vi "LinearSystemSim_setInput.vi"(9 "Battery_Volts":dbl=12.0, 10 "Input":T1, 11 "in LinearSystemSim":T2) -> (0 "Size Coerced":bool, 3 "out LinearSystemSim":T2)   [LabVIEW 2019, in "Trajectory_Library.lvlib"]
doc: "Sets the system inputs (usually voltages).\n \nInputs:\n - LinearSystemSim -- Data cluster\n - Input -- The system inputs (u).\n - BatteryVolts -- Current battery voltage (volts)\n\nOutputs:\n - OutLinearSystemSim -- Updated data cluster\n - SizeCoerced -- If TRUE, an error occured. Execution may continue."
uses:
  Trajectory_Library.lvlib
  TypeDef/LINEAR_SYSTEM.ctl
  <vilib>/Analysis/Matrix/Datatypes/RealMatrix.ctl
  <vilib>/Analysis/Matrix/NI_Matrix.lvlib
  TypeDef/LINEAR_SYSTEM_SIM.ctl
panel:
  # "<States, 1>"
  # "<Outputs, 1>"
  # "<Inputs, 1>"
  # "<Outputs, 1>"
  # "<States,States>"
  # "<States,Inputs>"
  # "<Outputs,States>"
  # "<Outputs,Inputs>"
  # "<States, 1>"
  # "<Outputs, 1>"
  # "<Inputs, 1>"
  # "<Outputs, 1>"
  # "<States,States>"
  # "<States,Inputs>"
  # "<Outputs,States>"
  # "<Outputs,Inputs>"
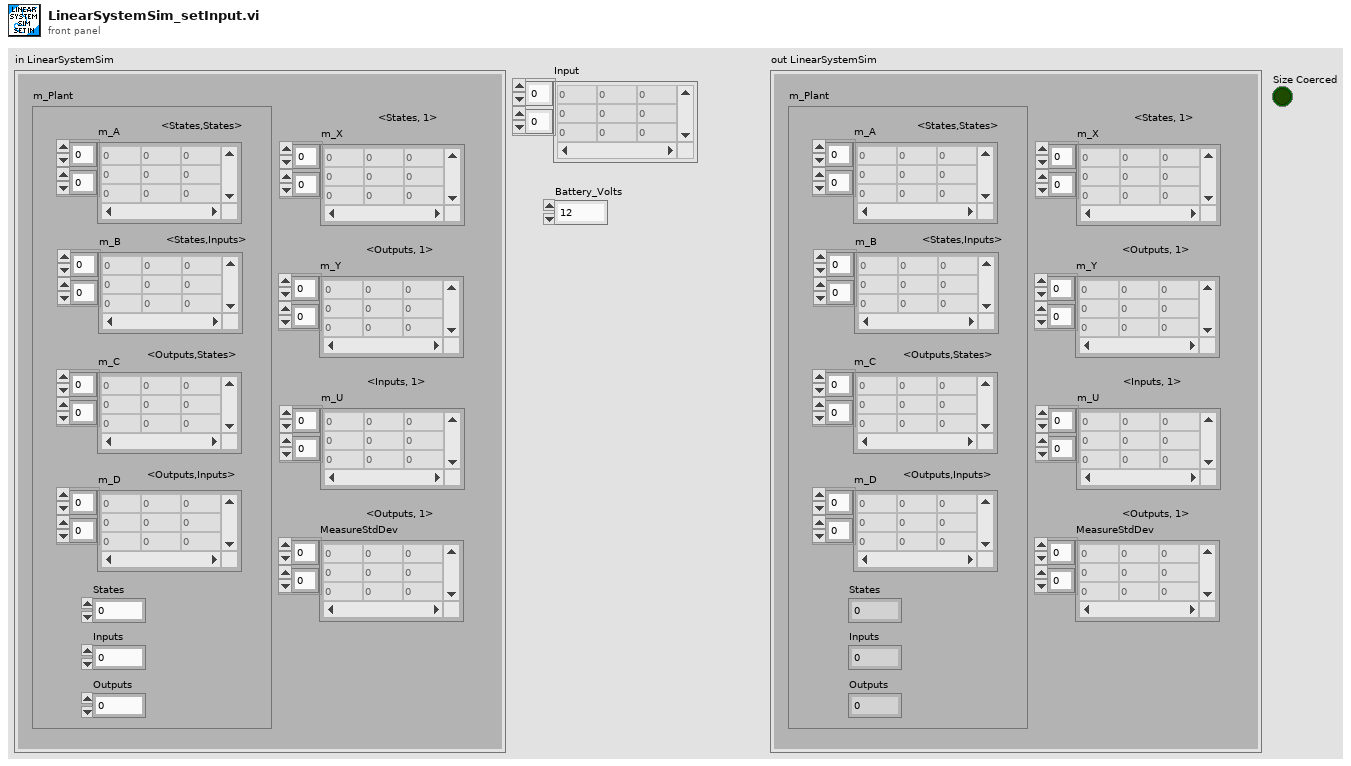
[diagram p1: front panel]
types:
  T1 = typedef "NI_Matrix.lvlib/RealMatrix.ctl" = dbl[][]
  T2 = typedef "Trajectory_Library.lvlib/LINEAR_SYSTEM_SIM.ctl" = cluster{"m_Plant":T3, "m_X":T1, "m_Y":T1, "m_U":T1, "MeasureStdDev":T1}
  T3 = typedef "Trajectory_Library.lvlib/LINEAR_SYSTEM.ctl" = cluster{"m_A":T1, "m_B":T1, "m_C":T1, "m_D":T1, "States":i32, "Inputs":i32, "Outputs":i32}
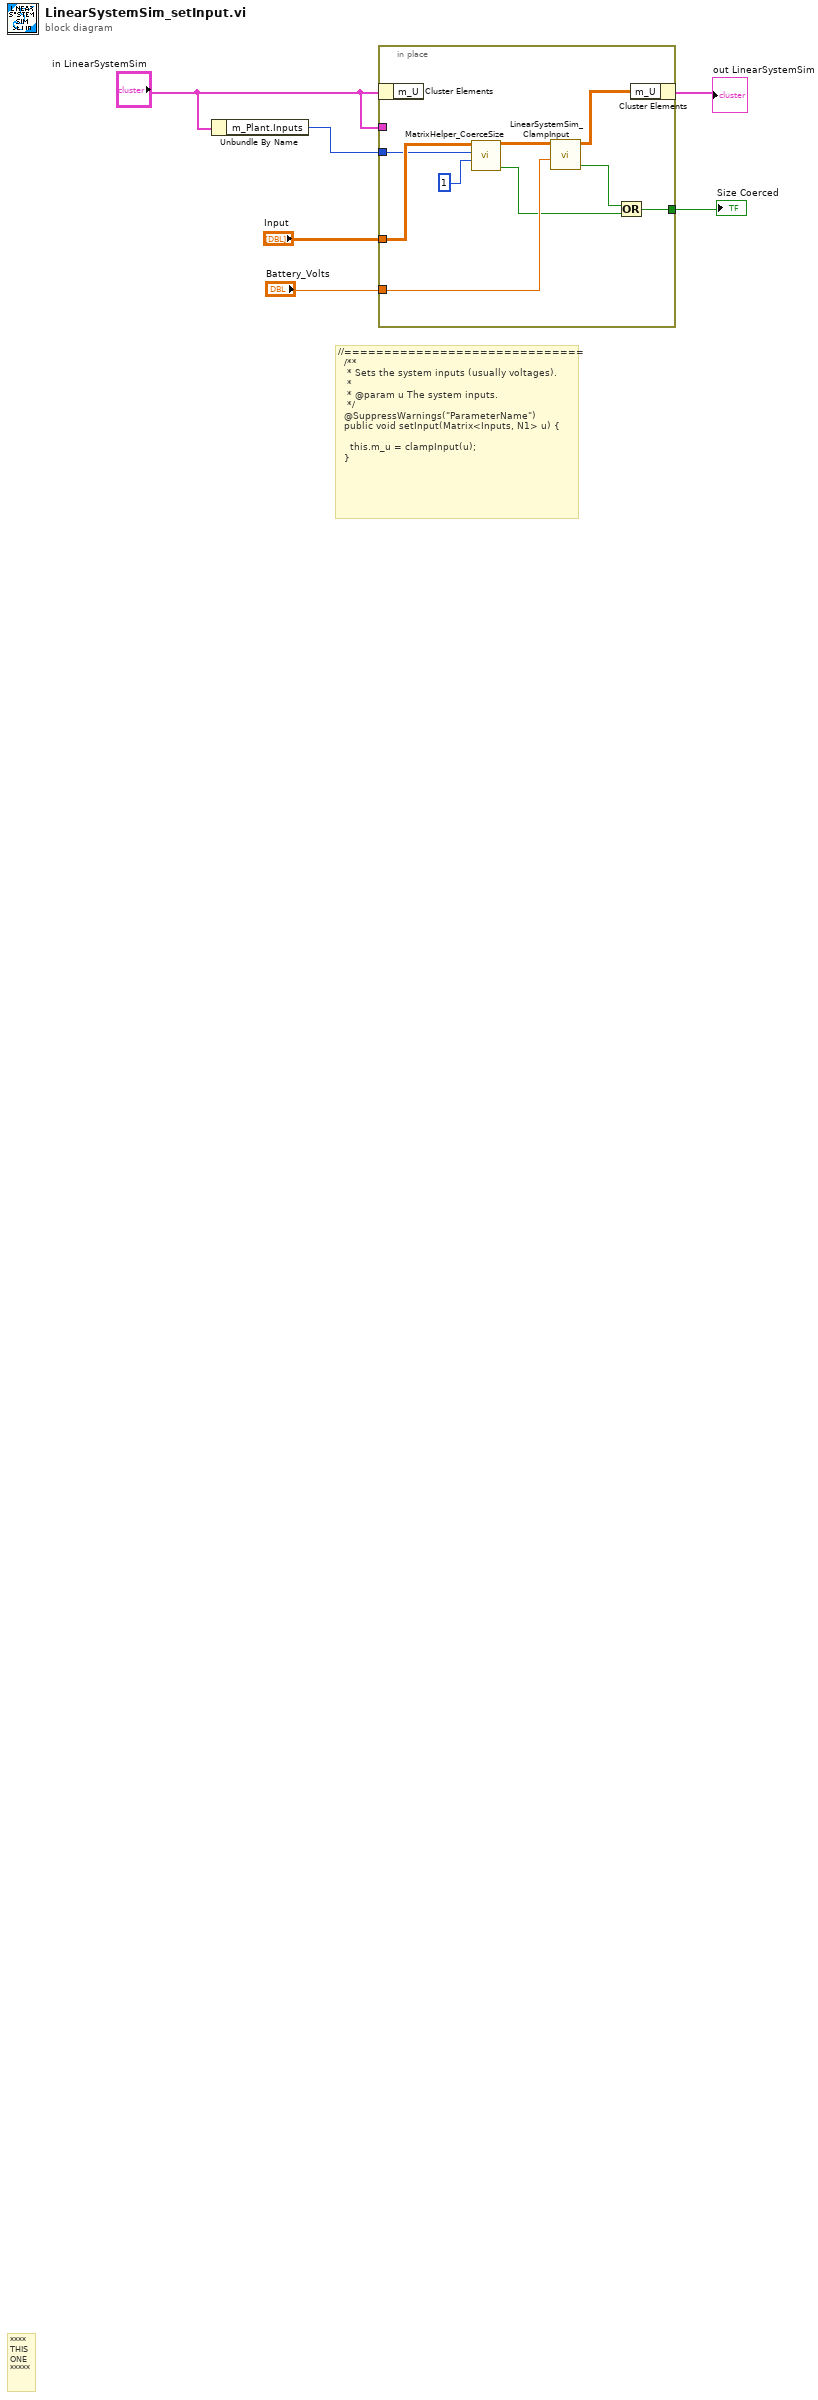
[diagram p0: block diagram]
diagram:
  # "//==============================\n  /**\n   * Sets the system inputs (usually voltages).\n   *\n   * @param u The system inputs.\n   */\n  @SuppressWarnings(\"ParameterName\")\n  public void setInput(Matrix<Inputs, N1> u) {\n\n    this.m_u = clampInput(u);\n  }"
  # "****\nTHIS\nONE\n*****"
  n1 = Unbundle By Name("in LinearSystemSim") -> ("m_Plant.Inputs"=w4:i32)
  n2 = in-place {
    in-place-border: "Input" -> [w15]
    in-place-border: w4 -> [w13]
    in-place-border: "in LinearSystemSim" -> [_]
    in-place-border: "Battery_Volts" -> [w10]
    in-place-border: [w7] -> w1
    n3 = in-place-cluster #1("in LinearSystemSim") -> ()  [unwired: 1 out]
    n4 = call "MatrixHelper_CoerceSize.vi"("Columns"=1, "Rows"=w13, "input matrix"=w15) -> ("Coerced"=w8:bool, "output matrix"=w11:T1)  [unwired: 7 in]
    n5 = call "LinearSystemSim_ClampInput.vi"("Battery_Volts"=w10, "Input"=w11) -> ("Size Coerced"=w9:bool, "ClampedInput"=w12:T1)  [unwired: 8 in]
    n6 = Or(x=w9, y=w8) -> (x .or. y?=w7:bool)
    n7 = in-place-cluster #1("m_U"=w12) -> (→"out LinearSystemSim":T2)
  }
  "Size Coerced" <- w1
